vi "Query Platform System Light.vi"(8 "error in (no error)":errorcluster, 11 "VISA resource name":refnum<visa-resource-name>) -> (0 "error out":errorcluster, 2 "Light State Enabled":bool, 3 "VISA resource name out":refnum<visa-resource-name>)   [LabVIEW 2018, in "LTB-1.lvlib" / "3150.lvlib"]
doc: "Queries the status of the light of instrument over interface."
uses:
  3150.lvlib
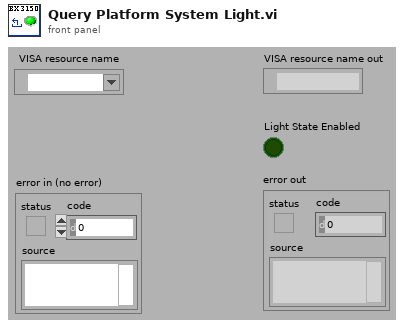
[diagram p1: front panel]
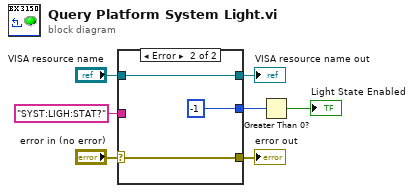
[diagram p0: block diagram]
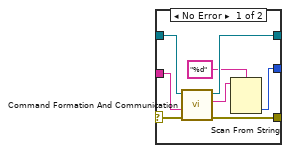
[diagram p2: hidden frame]
diagram:
  n1 = case shown="Error" "error in (no error)" {
    selector: "error in (no error)" -> [w14 w18]
    tunnel: [w13 w17] -> w5
    tunnel: "SYST:LIGH:STAT?" ("Command") -> [w15 _]
    tunnel: [w12 w18] -> w3
    tunnel: "VISA resource name" -> [w10 w17]
    tunnel: [w8 i16 -1] -> w2
    frame No Error {
      n2 = call "Command Formation And Communication.vi"("error in (no error)"=w14, "Command"=w15, "VISA resource name"=w10) -> ("error out"=w12:errorcluster, "Response"=w11:string, "VISA resource name out"=w13:refnum<visa-resource-name>)  [unwired: 1 in, 5 out]
      n3 = Scan From String(format string="%d", input string=w11) -> (output 1=w8:i32)  [unwired: 2 in, 4 out]
    }
    frame Error {
    }
  }
  "VISA resource name out" <- w5
  "error out" <- w3
  n4 = Greater Than 0?(x=w2) -> (x > 0?=→"Light State Enabled":bool)
